vi "Frame Color Write.vi"(4 "error in (no error)":errorcluster, 5 "Value":u32, 6 "Container State":T2, 7 "Display State In":T1={"Color 1"=0, "Color 2"=0, "Direction"=enum."Top to Bottom", "Frame Color"=16777216, "Fraction"=0.0}) -> (0 "error out":errorcluster, 3 "Display State Out":T1={"Color 1"=0, "Color 2"=0, "Direction"=enum."Top to Bottom", "Frame Color"=16777216, "Fraction"=0.0})   [LabVIEW 2020, in "KBackground Gradient.xctl"]
uses:
  KBackground Gradient.xctl
  <vilib>/_xctls/Container State.ctl
  State.vi
  <vilib>/_xctls/XControlSupport.lvlib
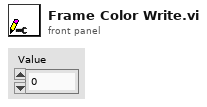
[diagram p1: front panel]
types:
  T1 = typedef "KBackground Gradient.xctl/State.vi" = cluster{"Color 1":u32, "Color 2":u32, "Direction":enum16{"Top to Bottom", "Bottom to Top", "Left to Right", "Right to Left"}, "Frame Color":u32, "Fraction":dbl}
  T2 = typedef "XControlSupport.lvlib/Container State.ctl" = cluster{"Indicator?":bool, "Run Mode?":bool, " Refnum":refnum<vi>}
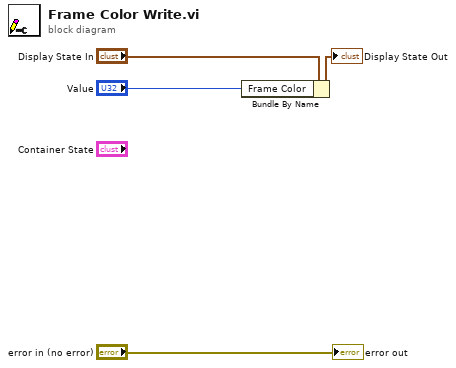
[diagram p0: block diagram]
diagram:
  n1 = Bundle By Name(cluster="Display State In", "Frame Color"="Value") -> (→"Display State Out":T1)
  "error out" <- "error in (no error)"
